vi "MDrive_Motor Log.vi"(6 "Motor Name":string, 7 "Function":string, 8 "Error in":errorcluster, 9 "read buffer":string, 10 "Param":string, 11 "COM":string) -> (0 "Error out":errorcluster)   [LabVIEW 2015]
uses:
  <vilib>/Utility/error.llb/DialogType.ctl
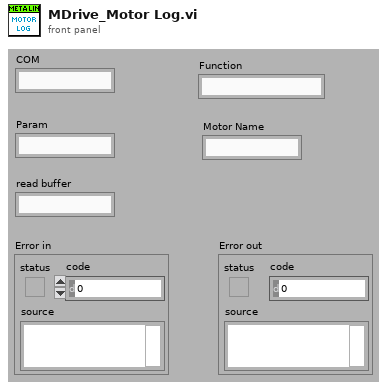
[diagram p1: front panel]
types:
  T1 = enum16{"open", "replace", "create", "open or create", "replace or create", "replace or create with confirmation"}
  T2 = typedef "DialogType.ctl" = u16
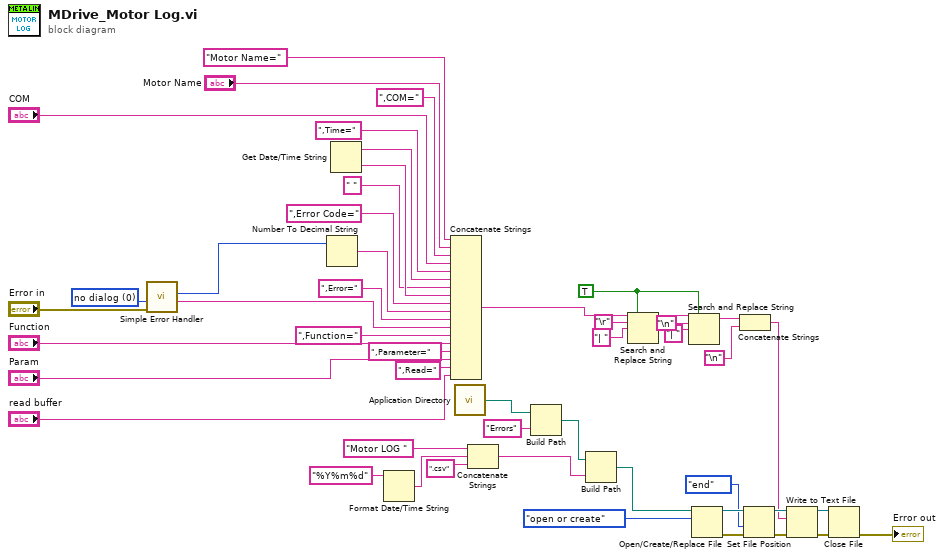
[diagram p0: block diagram]
diagram:
  w11 = TRUE ("replace all? (F)")
  w26 = T2 0 items=["no dialog", "OK message", "continue or stop message", "OK message + warnings", "continue/stop + warnings"] ("type of dialog (OK msg:1)")
  n1 = call <vilib>:"Simple Error Handler.vi"("type of dialog (OK msg:1)"=w26, "error in (no error)"="Error in") -> ("code out"=w24:i32, "source out"=w23:string)  [unwired: 3 in, 3 out]
  n2 = Number To Decimal String(number=w24) -> (decimal integer string=w40:string)  [unwired: 1 in]
  n3 = Get Date/Time String() -> (date string=w28:string, time string=w35:string)  [unwired: 3 in]
  n4 = Format Date/Time String(time format string (%c)="%Y%m%d") -> (date/time string=w37:string)  [unwired: 2 in]
  n5 = Concatenate Strings("Motor Name=" ("string"), "Motor Name", ",COM=" ("string"), "COM", ",Time=" ("string"), w28, " " ("string"), w35, ",Error Code=" ("string"), w40, ",Error=" ("string"), w23, ",Function=" ("string"), "Function", ",Parameter=" ("string"), "Param", ",Read=" ("string"), "read buffer") -> (w15:string)
  n6 = call <vilib>:"Application Directory.vi"() -> ("Application Directory"=w3:path)
  n7 = Concatenate Strings("Motor LOG " ("name or relative path"), w37, ".csv" ("string")) -> (w43:string)
  n8 = Build Path(base path=w3, name or relative path="Errors") -> (appended path=w1:path)
  n9 = Build Path(base path=w1, name or relative path=w43) -> (appended path=w45:path)
  n10 = Search and Replace String(replace all?=w11, input string=w15, search string="\r", replace string="| " ("replace string (\"\")")) -> (result string=w12:string)  [unwired: 4 in, 3 out]
  n11 = Search and Replace String(replace all?=w11, input string=w12, search string="\n", replace string="| " ("replace string (\"\")")) -> (result string=w8:string)  [unwired: 4 in, 3 out]
  n12 = Open/Create/Replace File(file path (use dialog)=w45, operation (0:open)=T1."open or create") -> (refnum out=w32:refnum<file>, error out=w46:errorcluster)  [unwired: 4 in, 1 out]
  n13 = Concatenate Strings(w8, "\n") -> (w6:string)
  n14 = Set File Position(refnum=w32, from (0:start)=enum16{"start", "end", "current"}."end", error in=w46) -> (refnum out=w31:refnum<file>, error out=w33:errorcluster)  [unwired: 1 in]
  n15 = Write to Text File(file (use dialog)=w31, text=w6, error in=w33) -> (refnum out=w48:refnum<file>, error out=w47:errorcluster)  [unwired: 1 in, 1 out]
  n16 = Close File(refnum=w48, error in=w47) -> (error out=→"Error out":errorcluster)  [unwired: 1 out]
